vi "Do Write.vi"(8 "error in (no error)":errorcluster, 10 "Interface":refnum<class "Interface.lvclass">, 11 "Section 1 in":refnum<class "Section 1.lvclass">) -> (0 "error out":errorcluster, 3 "Section 1 out":refnum<class "Section 1.lvclass">, 4 "All Keys Found?":bool)   [LabVIEW 2015, in "LVOOP Introduction.lvlib" / "Section 1.lvclass"]
doc: "Write keys/value pairs to Interface.\n\nOverwriting dynamic dispatch VI."
uses:
  Section 1.lvclass
  Configuration/Classes/Interface/Interface.lvclass
  Section 1.lvclass/Section 1.ctl
  Configuration/Classes/Section/Section.lvclass
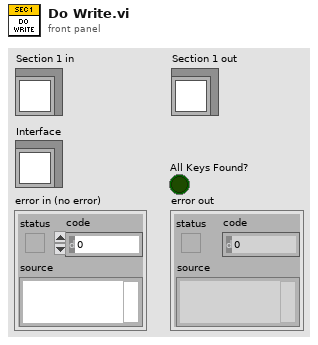
[diagram p1: front panel]
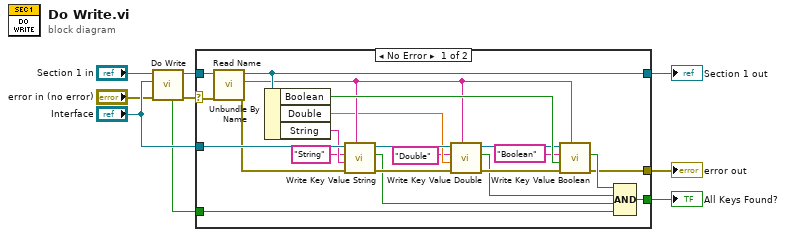
[diagram p0: block diagram]
diagram:
  n1 = call-parent "Do Write.vi"("error in (no error)"="error in (no error)", "Interface"="Interface", "Section in"="Section 1 in") -> ("error out"=w2:errorcluster, "Section out"=w5:refnum<class "Section 1.lvclass">, "All Keys Found?"=w1:bool)  [unwired: 6 in]
  n2 = case shown="No Error" w2 {
    selector: w2 -> [w11 w32]
    tunnel: w5 -> [w12 w33]
    tunnel: "Interface" -> [w30 _]
    tunnel: [w27 w33] -> w9
    tunnel: [w15 _] -> w8
    tunnel: [w13 w32] -> w7
    tunnel: w1 -> [w10 _]
    frame No Error {
      n3 = call "Read Name.vi"("error in (no error)"=w11, "Section in"=w12) -> ("error out"=w14:errorcluster, "Name"=w26:string, "Section out"=w27:refnum<class "Section 1.lvclass">)  [unwired: 7 in]
      n4 = Unbundle By Name(w27) -> ("Boolean"=w31:bool, "Double"=w25:dbl, "String"=w24:string)
      n5 = call-dynamic "Write Key Value String.vi"("Section Name"=w26, "error in (no error)"=w14, "Value"=w24, "Key Name"="String", "Interface in"=w30) -> ("error out"=w20:errorcluster, "found"=w16:bool, "Interface out"=w29:refnum<class "Interface.lvclass">)  [unwired: 4 in]
      n6 = call-dynamic "Write Key Value Double.vi"("Section Name"=w26, "error in (no error)"=w20, "Value"=w25, "Key Name"="Double", "Interface in"=w29) -> ("error out"=w19:errorcluster, "found"=w17:bool, "Interface out"=w28:refnum<class "Interface.lvclass">)  [unwired: 4 in]
      n7 = call-dynamic "Write Key Value Boolean.vi"("Section Name"=w26, "error in (no error)"=w19, "Value"=w31, "Key Name"="Boolean", "Interface in"=w28) -> ("error out"=w13:errorcluster, "found"=w18:bool)  [unwired: 4 in, 1 out]
      n8 = Compound Arithmetic op=AND(w18, w17, w16, w10) -> (w15:bool)
    }
    frame Error {
    }
  }
  "error out" <- w7
  "Section 1 out" <- w9
  "All Keys Found?" <- w8
